vi "VS-Read Temp.vi"(8 "error in (no error)":errorcluster) -> (0 "error out":errorcluster, 2 "Temp (C)":dbl format="%.1f")   [LabVIEW 2020]
uses:
  <vilib>/Utility/sysdir.llb/System Directory Type.ctl
  Typedefs/PhysMon-Options.ctl
  Typedefs/PhysMon-Scale.ctl
  Typedefs/PhysMon-TempSensor.ctl
  Typedefs/PhysMon-HR From EKG Settings.ctl
  Connection Manager/Type Defs/Input sources.ctl
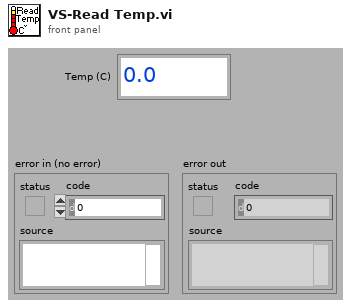
[diagram p1: front panel]
types:
  T1 = typedef "Input sources.ctl" = u16
  T2 = typedef "PhysMon-Options.ctl" = cluster{"Min Interval":dbl, "HR from ABR?":bool, "HR Scale":T3, "Temp Scale":T3, "Lock?":bool, "Temp Sensor":T4, "EKG":T5}
  T3 = typedef "PhysMon-Scale.ctl" = cluster{"Slope":dbl, "Offset":dbl, "Limits":cluster{"Min":dbl, "Max":dbl}, "term config":i32}
  T4 = typedef "PhysMon-TempSensor.ctl" = enum16{"YSI", "FHC", "Custom"}
  T5 = typedef "PhysMon-HR From EKG Settings.ctl" = cluster{"Sample duration (s)":dbl}
  T6 = typedef "System Directory Type.ctl" = i32
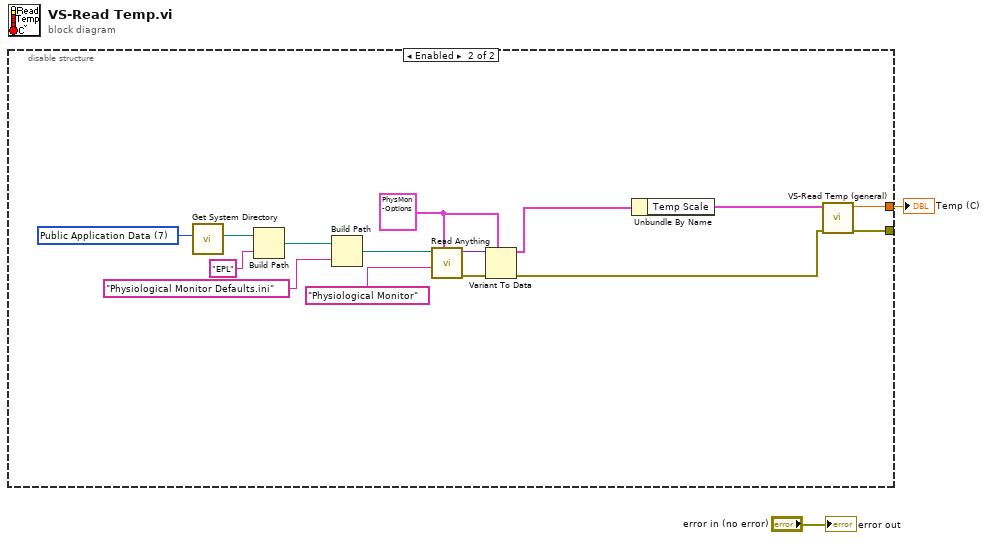
[diagram p0: block diagram]
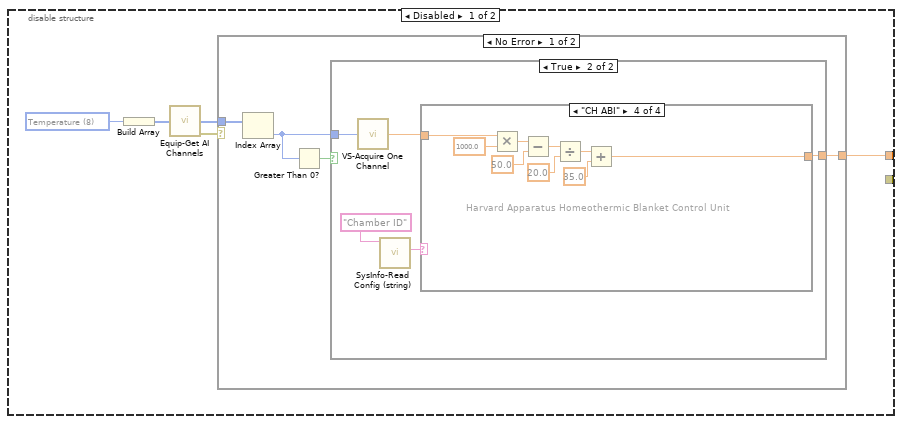
[diagram p2: hidden frame]
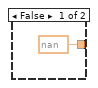
[diagram p3: hidden frame]
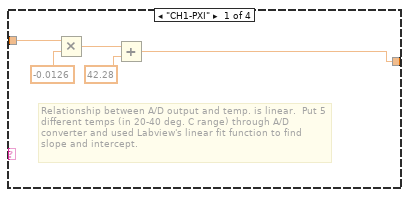
[diagram p4: hidden frame]
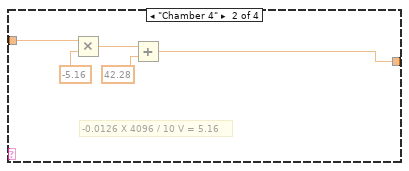
[diagram p5: hidden frame]
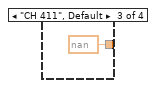
[diagram p6: hidden frame]
diagram:
  n1 = disable-structure shown="Enabled" {
    disable-tunnel: [w7 w47] -> w2
    disable-tunnel: [_ w38] -> _
    frame Disabled {
      w6 = T1 8 items=["--unused--", "Probe Mic Right", "Probe Mic Left", "Cal Mic", "ABR", "CAP Right", "CAP Left", "Startle piezo", "Temperature", "Heart rate"] ("Ring")
      n2 = Build Array(w6) -> (w5:T1[])
      n3 = call "Equip-Get AI Channels.vi"("Inputs"=w5) -> ("AI Channels"=w4:i32[], "error out"=w3:errorcluster)  [unwired: 13 in]
      n4 = case shown="No Error" w3 {
        tunnel: [w11 _] -> w7
        tunnel: w4 -> [w10 _]
        frame No Error {
          n5 = Index Array(array=w10) -> (element=w9:i32)  [unwired: 1 in]
          n6 = Greater Than 0?(x=w9) -> (x > 0?=w8:bool)
          n7 = case shown="True" w8 {
            tunnel: [nan w17] -> w11
            tunnel: w9 -> [_ w15]
            frame False {
            }
            frame True {
              n8 = call "VS-Acquire One Channel.vi"("index"=w15) -> ("mean"=w16:dbl)  [unwired: 13 in, 1 out]
              n9 = call "SysInfo-Read Config (string).vi"("key"="Chamber ID" ("string")) -> ("value"=w13:string)  [unwired: 8 in, 2 out]
              n10 = case shown="\"CH ABI\"" w13 {
                tunnel: w16 -> [w22 w24 _ w30]
                tunnel: [w18 w23 nan w29] -> w17
                frame "CH1-PXI" {
                  # "Relationship between A/D output and temp. is linear.  Put 5 different temps (in 20-40 deg. C range) through A/D converter and used Labview's linear fit function to find slope and intercept."
                  n11 = Multiply(x=w22, y=-0.0126) -> (x*y=w20:dbl)
                  n12 = Add(x=w20, y=42.28) -> (x+y=w18:dbl)
                }
                frame "Chamber 4" {
                  # "-0.0126 X 4096 / 10 V = 5.16"
                  n13 = Multiply(x=w24, y=-5.16) -> (x*y=w26:dbl)
                  n14 = Add(x=w26, y=42.28) -> (x+y=w23:dbl)
                }
                frame "CH 411", Default {
                }
                frame "CH ABI" {
                  # "Harvard Apparatus Homeothermic Blanket Control Unit"
                  n15 = Multiply(x=w30, y=1000.0) -> (x*y=w32:dbl)
                  n16 = Subtract(x=w32, y=50.0) -> (x-y=w34:dbl)
                  n17 = Divide(x=w34, y=20.0) -> (x/y=w36:dbl)
                  n18 = Add(x=w36, y=35.0) -> (x+y=w29:dbl)
                }
              }
            }
          }
        }
        frame Error {
        }
      }
    }
    frame Enabled {
      w43 = T2 {"Min Interval"=0.0, "HR from ABR?"=FALSE, "HR Scale"={"Slope"=0.0, "Offset"=0.0, "Limits"={"Min"=0.0, "Max"=0.0}, "term config"=-1}, "Temp Scale"={"Slope"=0.0, "Offset"=0.0, "Limits"={"Min"=0.0, "Max"=0.0}, "term config"=-1}, "Lock?"=FALSE, "Temp Sensor"=enum."YSI", "EKG"={"Sample duration (s)"=0.0}} ("Options")
      w52 = T6 7 items=["User Home", "User Desktop", "User Documents", "User Application Data", "User Preferences", "User Temporary", "Public Documents", "Public Application Data", "Public Preferences", "System Core Libraries", "System Installed Libraries", "Application Files", "Boot Volume Root"] ("system directory type")
      n19 = call <vilib>:"Get System Directory.vi"("system directory type"=w52) -> ("system directory"=w51:path)  [unwired: 10 in]
      n20 = Build Path(base path=w51, name or relative path="EPL") -> (appended path=w49:path)
      n21 = Build Path(base path=w49, name or relative path="Physiological Monitor Defaults.ini") -> (appended path=w45:path)
      n22 = call "Read Anything.vi"("Type of Anything"=w43, "Section Name (Name of \"Type of Anything\")"="Physiological Monitor" ("Section Name (Name of \"Type of Anything\")"), "Path (dialog)"=w45) -> ("Error Out"=w41:errorcluster, "Anything"=w46:variant)  [unwired: 6 in, 1 out]
      n23 = Variant To Data(error in=w41, type=w43, Variant=w46) -> (data=w40:T2, error out=w42:errorcluster)
      n24 = Unbundle By Name(w40) -> ("Temp Scale"=w39:T3)
      n25 = call "VS-Read Temp (general).vi"("error in (no error)"=w42, "Scale"=w39) -> ("error out"=w38:errorcluster, "Temp (C)"=w47:dbl)  [unwired: 7 in, 1 out]
    }
  }
  "Temp (C)" <- w2
  "error out" <- "error in (no error)"
